vi "Instrument.vi"() -> ()   [LabVIEW 2019, in "Instrument.lvlib"]
uses:
  Instrument.lvlib
  MsgQ/TypeDefs/CommandsQ.ctl
  MsgQ/TypeDefs/MsgQ_Commands.ctl
  States.ctl
  Service/Service.lvlib
  MsgQ/MsgQ.lvlib
panel:
  out "# Recv'd commands":i32
  out "state":T1
  out "# iterations":i32
  in  "reset":bool
  out "CMDs":T2[](array[typedef])
  in  "stop":bool
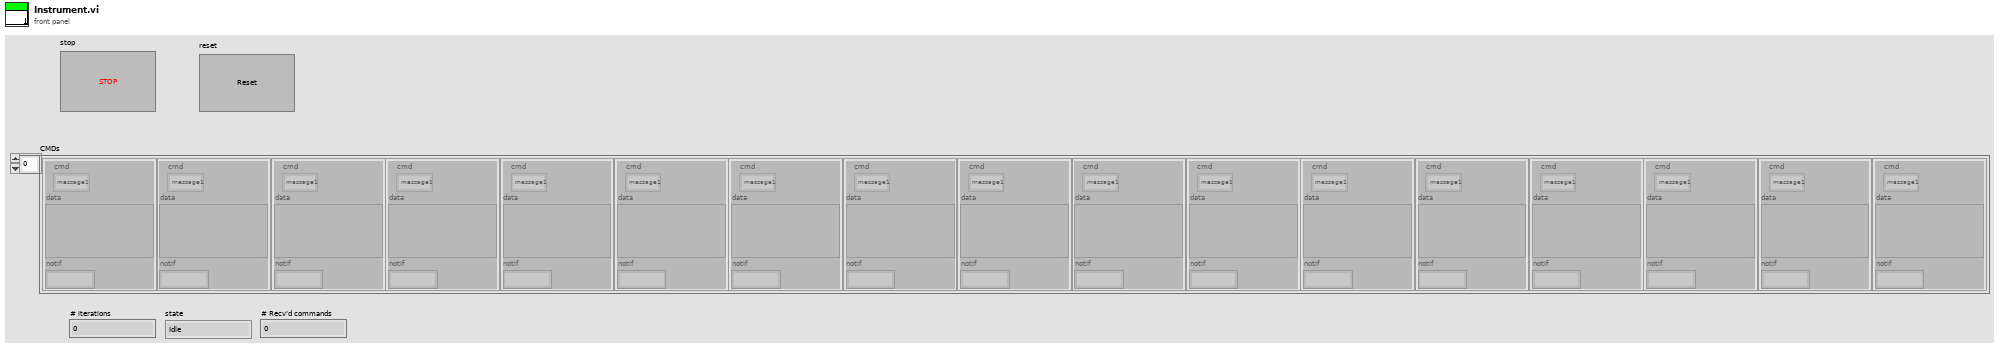
[diagram p1: front panel]
types:
  T1 = typedef "Service.lvlib/States.ctl" = enum16{"Idle", "Init", "PollMsgQ", "Shtudown"}
  T2 = typedef "Service.lvlib/CommandsQ.ctl" = cluster{"cmd":T3, "data":variant, "notif":string}
  T3 = typedef "MsgQ.lvlib/MsgQ_Commands.ctl" = enum16{"message1", "message2", "message3", "generic", "transparent", "exception", "stop"}
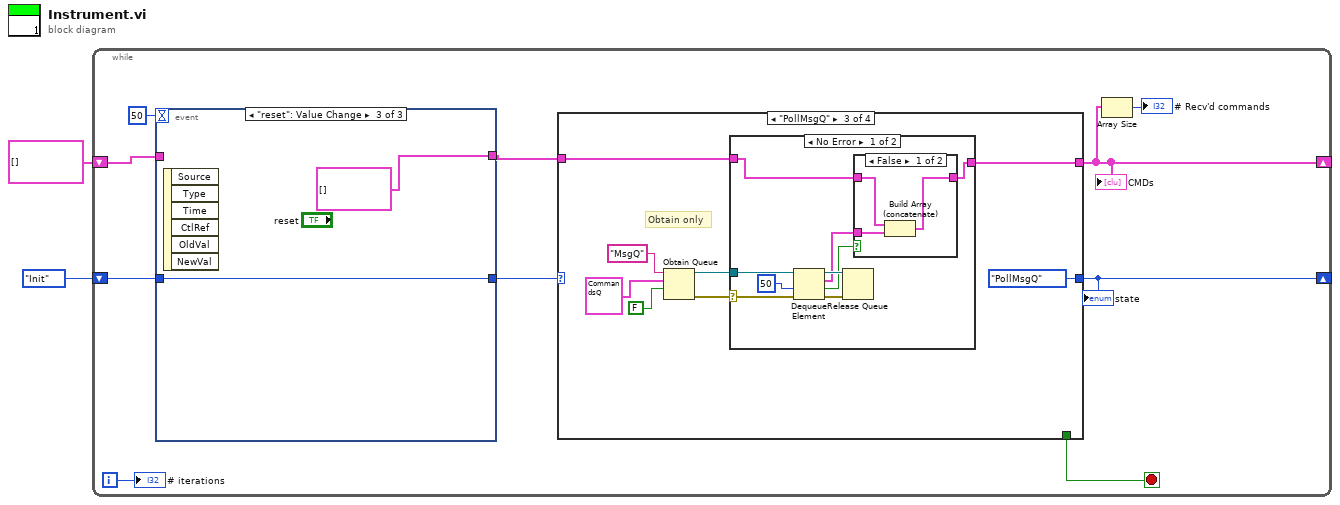
[diagram p0: block diagram]
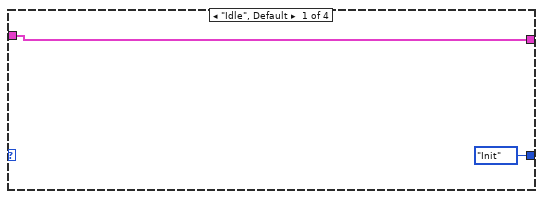
[diagram p2: hidden frame]
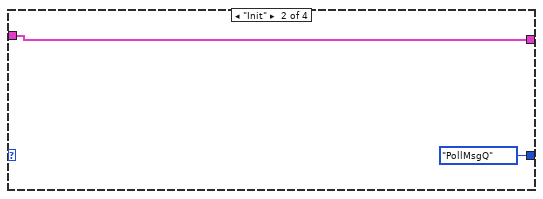
[diagram p3: hidden frame]
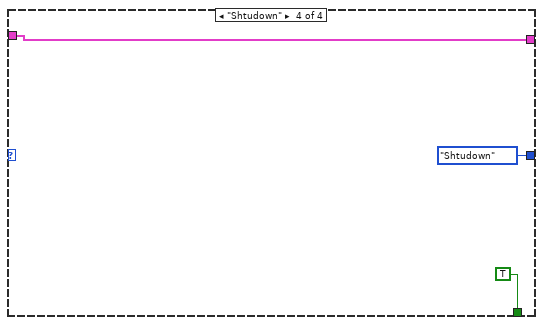
[diagram p6: hidden frame]
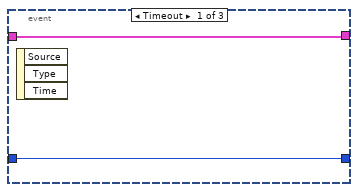
[diagram p7: hidden frame]
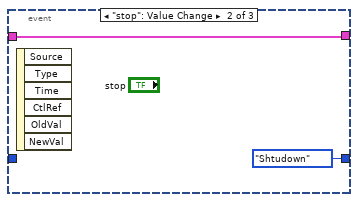
[diagram p8: hidden frame]
diagram:
  n1 = while {
    shift-right: [w10] -> _
    shift-left: States."Init" -> [w12]
    shift-right: [w4] -> _
    shift-left: T2[] [] -> [w8]
    i -> [w6]
    stop <- w9 stop-if-true
    n2 = event shown="[2] \"reset\": Value Change" {
      selector: _ -> [_ _ _]
      dyn-events: _ -> [_ _ _]
      timeout: 50 -> [_ _ _]
      tunnel: w12 -> [w43 _ w47]
      tunnel: [w43 States."Shtudown" w47] -> w11
      tunnel: w8 -> [w42 w44 _]
      tunnel: [w42 w44 T2[] []] -> w7
      event Timeout {
        n3 = event-data() -> ()  [unwired: 1 in, 3 out]
      }
      event "stop": Value Change {
        n4 = event-data() -> ()  [unwired: 1 in, 6 out]
      }
      event "reset": Value Change {
        n5 = event-data() -> ()  [unwired: 1 in, 6 out]
      }
    }
    n6 = case shown="\"PollMsgQ\"" w11 {
      tunnel: [States."Init" States."PollMsgQ" States."PollMsgQ" States."Shtudown"] -> w10
      tunnel: [_ _ _ TRUE] -> w9
      tunnel: [w14 w15 w17 w39] -> w4
      tunnel: w7 -> [w14 w15 w18 w39]
      frame "Idle", Default {
      }
      frame "Init" {
      }
      frame "PollMsgQ" {
        # "Obtain only"
        n7 = Obtain Queue(name (unnamed)="MsgQ", element data type=T2 {"cmd"=enum."message1", "data"=variant, "notif"="notif1"}, create if not found? (T)=FALSE) -> (queue out=w21:refnum<queue>, error out=w19:errorcluster)  [unwired: 2 in, 1 out]
        n8 = case shown="No Error" w19 {
          selector: w19 -> [w29 _]
          tunnel: w21 -> [w33 _]
          tunnel: w18 -> [w27 w38]
          tunnel: [w26 w38] -> w17
          frame No Error {
            n9 = Dequeue Element(queue=w33, timeout in ms (-1)=50, error in (no error)=w29) -> (queue out=w31:refnum<queue>, element=w28:T2, timed out?=w25:bool, error out=w30:errorcluster)
            n10 = Release Queue(queue=w31, error in (no error)=w30) -> ()  [unwired: 1 in, 3 out]
            n11 = case shown="False" w25 {
              tunnel: w28 -> [w36 _]
              tunnel: w27 -> [w35 w37]
              tunnel: [w34 w37] -> w26
              frame False {
                n12 = Build Array (concatenate)(w35, w36) -> (w34:T2[])
              }
              frame True {
              }
            }
          }
          frame Error {
          }
        }
      }
      frame "Shtudown" {
      }
    }
    "CMDs" <- w4
    "state" <- w10
    n13 = Array Size(array=w4) -> (size(s)=→"# Recv'd commands":i32)
    "# iterations" <- w6
  }
